vi "Motors Backlash.vi"(0 "X":u32, 1 "Y":u32, 2 "VISA in":refnum<visa-resource-name>, 3 "error in":errorcluster, 5 "Z":u32, 6 "Theta":u32) -> (7 "VISA out":refnum<visa-resource-name>, 9 "error out":errorcluster)   [LabVIEW 2018]
panel:
  out "read buffer Theta":string
  out "read buffer Z":string
  out "read buffer Y":string
  out "read buffer X":string
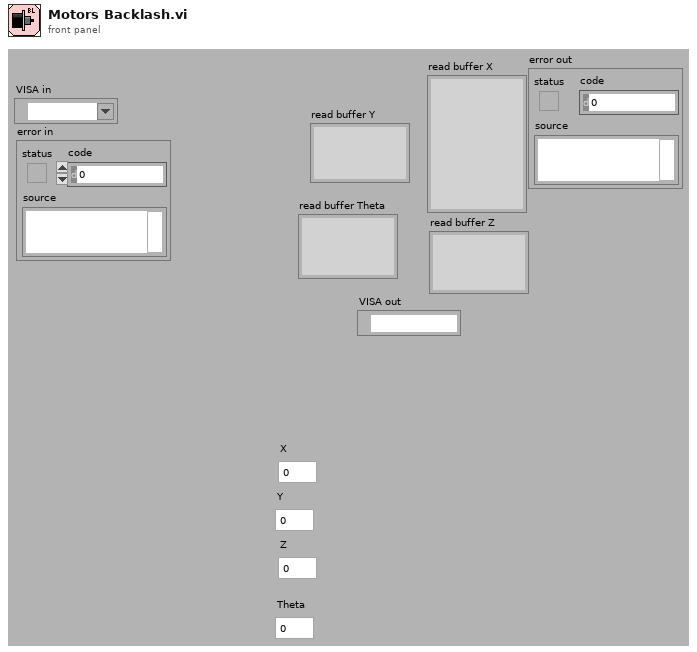
[diagram p1: front panel]
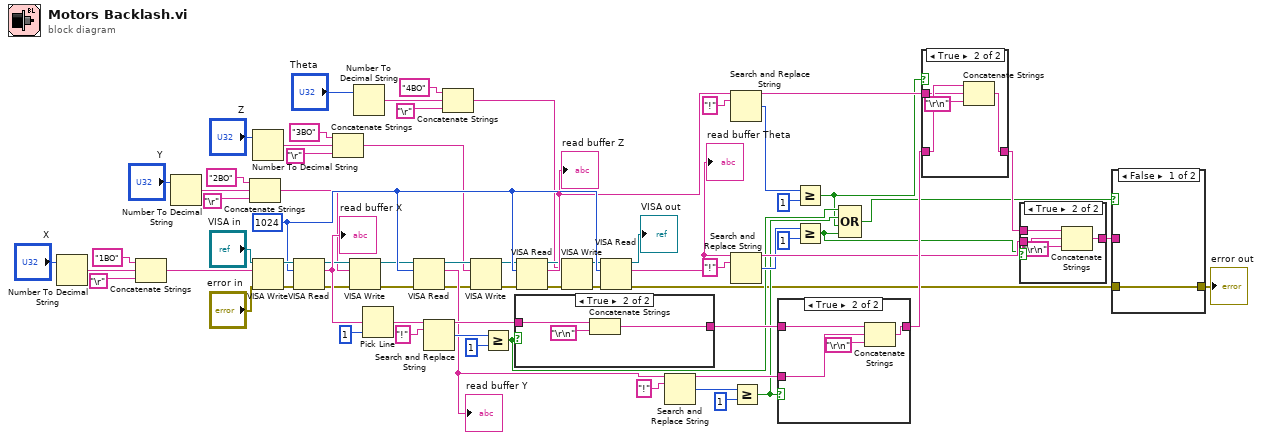
[diagram p0: block diagram]
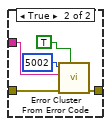
[diagram p2: hidden frame]
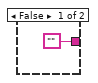
[diagram p6: hidden frame]
diagram:
  w69 = 1024
  n1 = Number To Decimal String(number="X") -> (decimal integer string=w46:string)  [unwired: 1 in]
  n2 = Concatenate Strings("1BO", w46, "\r") -> (w38:string)
  n3 = Number To Decimal String(number="Y") -> (decimal integer string=w44:string)  [unwired: 1 in]
  n4 = Concatenate Strings("2BO", w44, "\r") -> (w33:string)
  n5 = Number To Decimal String(number="Z") -> (decimal integer string=w42:string)  [unwired: 1 in]
  n6 = VISA Write(VISA resource name="VISA in", write buffer=w38, error in (no error)="error in") -> (VISA resource name out=w71:refnum<visa-resource-name>, error out=w70:errorcluster)  [unwired: 1 out]
  n7 = VISA Read(VISA resource name=w71, byte count=w69, error in (no error)=w70) -> (VISA resource name out=w34:refnum<visa-resource-name>, read buffer=w66:string, error out=w35:errorcluster)  [unwired: 1 out]
  "read buffer X" <- w66
  n8 = Concatenate Strings("3BO", w42, "\r") -> (w28:string)
  n9 = VISA Write(VISA resource name=w34, write buffer=w33, error in (no error)=w35) -> (VISA resource name out=w37:refnum<visa-resource-name>, error out=w36:errorcluster)  [unwired: 1 out]
  n10 = Number To Decimal String(number="Theta") -> (decimal integer string=w39:string)  [unwired: 1 in]
  n11 = Pick Line(multi-line string=w66, line index=1) -> (output string=w64:string)  [unwired: 1 in]
  n12 = VISA Read(VISA resource name=w37, byte count=w69, error in (no error)=w36) -> (VISA resource name out=w32:refnum<visa-resource-name>, read buffer=w61:string, error out=w30:errorcluster)  [unwired: 1 out]
  "read buffer Y" <- w61
  n13 = Search and Replace String(input string=w64, search string="!") -> (result string=w62:string, number of replacements=w63:i32)  [unwired: 6 in, 2 out]
  n14 = Concatenate Strings("4BO", w39, "\r") -> (w23:string)
  n15 = VISA Write(VISA resource name=w32, write buffer=w28, error in (no error)=w30) -> (VISA resource name out=w31:refnum<visa-resource-name>, error out=w29:errorcluster)  [unwired: 1 out]
  n16 = Greater Or Equal?(x=w63, y=1) -> (x >= y?=w14:bool)
  n17 = case shown="True" w14 {
    tunnel: w62 -> [_ w75]
    tunnel: ["" w74] -> w58
    frame False {
    }
    frame True {
      n18 = Concatenate Strings(w75, "\r\n") -> (w74:string)
    }
  }
  n19 = VISA Read(VISA resource name=w31, byte count=w69, error in (no error)=w29) -> (VISA resource name out=w25:refnum<visa-resource-name>, read buffer=w57:string, error out=w24:errorcluster)  [unwired: 1 out]
  "read buffer Z" <- w57
  n20 = VISA Write(VISA resource name=w25, write buffer=w23, error in (no error)=w24) -> (VISA resource name out=w27:refnum<visa-resource-name>, error out=w26:errorcluster)  [unwired: 1 out]
  n21 = VISA Read(VISA resource name=w27, byte count=w69, error in (no error)=w26) -> (VISA resource name out=→"VISA out":refnum<visa-resource-name>, read buffer=w53:string, error out=w8:errorcluster)  [unwired: 1 out]
  "read buffer Theta" <- w53
  n22 = Search and Replace String(input string=w61, search string="!") -> (result string=w59:string, number of replacements=w60:i32)  [unwired: 6 in, 2 out]
  n23 = Search and Replace String(input string=w57, search string="!") -> (result string=w54:string, number of replacements=w56:i32)  [unwired: 6 in, 2 out]
  n24 = Search and Replace String(input string=w53, search string="!") -> (result string=w51:string, number of replacements=w49:i32)  [unwired: 6 in, 2 out]
  n25 = Greater Or Equal?(x=w60, y=1) -> (x >= y?=w13:bool)
  n26 = case shown="True" w13 {
    tunnel: w59 -> [_ w79]
    tunnel: w58 -> [w76 w80]
    tunnel: [w76 w78] -> w55
    frame False {
    }
    frame True {
      n27 = Concatenate Strings(w80, w79, "\r\n") -> (w78:string)
    }
  }
  n28 = Greater Or Equal?(x=w56, y=1) -> (x >= y?=w12:bool)
  n29 = Greater Or Equal?(x=w49, y=1) -> (x >= y?=w11:bool)
  n30 = Compound Arithmetic op=OR(w14, w13, w12, w11) -> (w10:bool)
  n31 = case shown="True" w12 {
    tunnel: w55 -> [w81 w85]
    tunnel: w54 -> [_ w84]
    tunnel: [w81 w83] -> w48
    frame False {
    }
    frame True {
      n32 = Concatenate Strings(w85, w84, "\r\n") -> (w83:string)
    }
  }
  n33 = case shown="True" w11 {
    tunnel: w51 -> [_ w89]
    tunnel: w48 -> [w86 w90]
    tunnel: [w86 w88] -> w9
    frame False {
    }
    frame True {
      n34 = Concatenate Strings(w90, w89, "\r\n") -> (w88:string)
    }
  }
  n35 = case shown="False" w10 {
    tunnel: w9 -> [_ w96]
    tunnel: w8 -> [w91 w93]
    tunnel: [w91 w92] -> w7
    frame False {
    }
    frame True {
      n36 = call <vilib>:"Error Cluster From Error Code.vi"("show call chain? (False)"=TRUE, "error in (no error)"=w93, "error message (\"\")"=w96, "error code (0)"=5002) -> ("error out"=w92:errorcluster)  [unwired: 5 in]
    }
  }
  "error out" <- w7
